vi "DriverStation Get Remaining Match Time.vi"(8 "error in (no error)":errorcluster) -> (0 "error out":errorcluster, 2 "OutputsEnabled?":bool, 3 "Match Time(s)":sgl)   [LabVIEW 2026, in "MrcLib.lvlib"]
doc: "Returns the time remaining in the current portion of the robot match. It returns -1 if the robot is disabled or in an untimed mode."
uses:
  MrcLib.lvlib
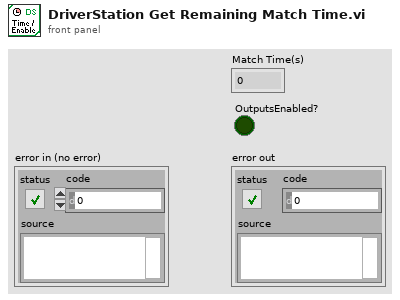
[diagram p1: front panel]
types:
  T1 = typedef "MrcLib.lvlib/MRC_ControlData.ctl" = cluster{"controlFlags":u32, "matchTime":u16, "currentOpMode":u64, "gameDataLength":u8, "gameData":cluster{"gameData 0":u8, "gameData 1":u8, "gameData 2":u8, "gameData 3":u8, "gameData 4":u8, "gameData 5":u8, "gameData 6":u8, "gameData 7":u8}}
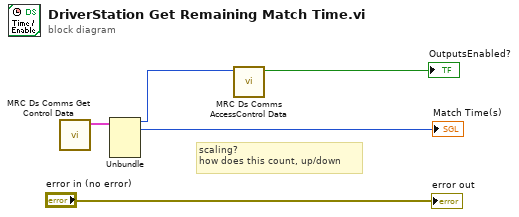
[diagram p0: block diagram]
diagram:
  # "scaling?\nhow does this count, up/down"
  n1 = call "MRC Ds Comms Get Control Data.vi"() -> ("data out"=w4:T1)  [unwired: 10 in, 1 out]
  n2 = Unbundle(w4) -> ("controlFlags"=w1:u32, "matchTime"=→"Match Time(s)":u16)  [unwired: 3 out]
  n3 = call "MRC Ds Comms AccessControl Data.vi"("controlFlag"=w1) -> ("Enabled"=→"OutputsEnabled?":bool)  [unwired: 7 in, 3 out]
  "error out" <- "error in (no error)"
